vi "FA_ReadXML.vi"(6 "Error In":errorcluster, 8 "Special Type":T1) -> (0 "Error Out":errorcluster, 2 "XML String":string)   [LabVIEW 2014, in "FA_LocalStore.lvlib"]
doc: "Returns the XML from LocalStore for a given Special Type."
uses:
  FA_LocalStore.lvlib
  FA_LSSpecialTypes.ctl
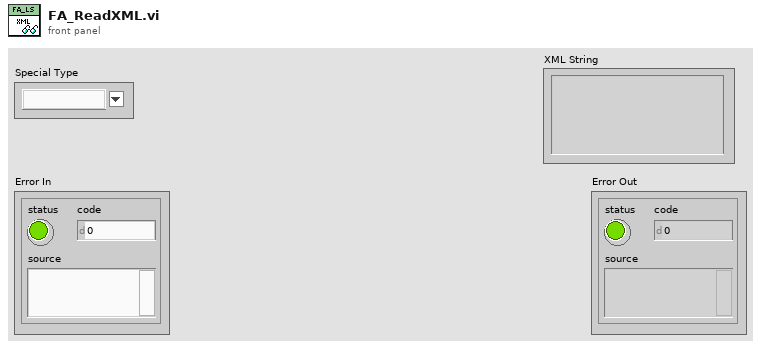
[diagram p1: front panel]
types:
  T1 = typedef "FA_LocalStore.lvlib/FA_LSSpecialTypes.ctl" = string
  T2 = typedef "FA_LocalStore.lvlib/FA_LSRef.ctl" = cluster{"eTag INI Refnum":T3, "XML Refnum Array":refnum<file>[]}
  T3 = typedef "NI_LVConfig.lvlib/Config Data RefNum.ctl" = refnum<k1>
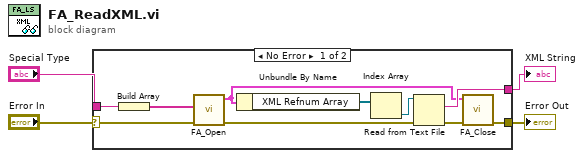
[diagram p0: block diagram]
diagram:
  n1 = case shown="No Error" "Error In" {
    selector: "Error In" -> [w11 w15]
    tunnel: [w6 w15] -> w4
    tunnel: "Special Type" -> [w10 _]
    tunnel: [w14 _] -> w2
    frame No Error {
      n2 = Build Array(w10) -> (w9:T1[])
      n3 = call "FA_Open.vi"("Error In"=w11, "Special Types Array"=w9) -> ("Error Out"=w5:errorcluster, "FA_LS Ref"=w8:T2)  [unwired: 8 in]
      n4 = Unbundle By Name(w8) -> ("XML Refnum Array"=w13:refnum<file>[])
      n5 = Index Array(array=w13) -> (element=w12:refnum<file>)  [unwired: 1 in]
      n6 = Read from Text File(file (use dialog)=w12, error in=w5) -> (text=w14:string, error out=w7:errorcluster)  [unwired: 2 in, 2 out]
      n7 = call "FA_Close.vi"("Error In"=w7, "FA_LS Ref"=w8) -> ("Error Out"=w6:errorcluster)  [unwired: 9 in]
    }
    frame Error {
    }
  }
  "Error Out" <- w4
  "XML String" <- w2
